vi "led_globals.vi"() -> ()   [LabVIEW 2021]
panel:
  in  "Button":bool
  out "LED":bool
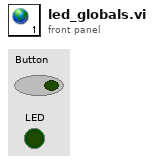
[diagram p1: front panel]
diagram:
